vi "WF0_RLE_griffin.vi"(0 "connection ID in":refnum<k5>, 1 "TxPulseRleA":string, 2 "Mode control":enum32{"D-mode", "B-mode"}(ring), 3 "Timeout (ms)":i32=40000000, 4 "TxFrequencyIndex":i8) -> (5 "connection ID out":refnum<k5>, 7 "Timeout (ms) out":i32)   [LabVIEW 2016]
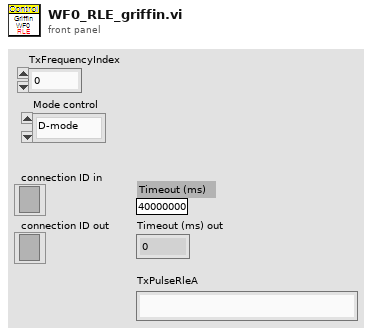
[diagram p1: front panel]
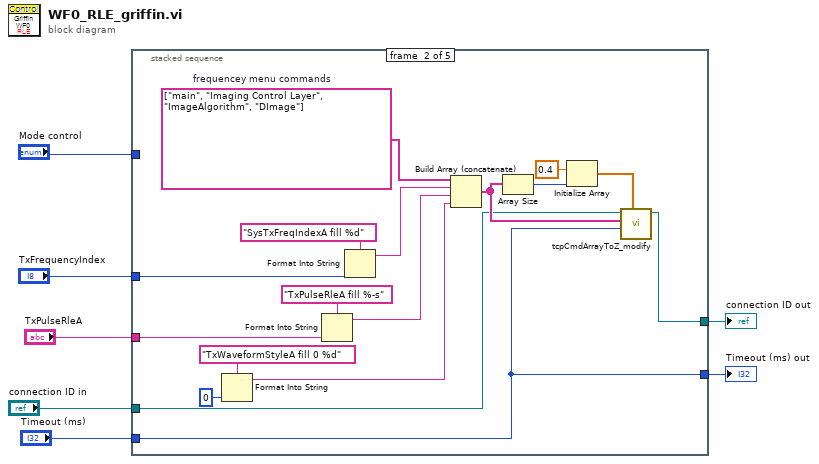
[diagram p0: block diagram]
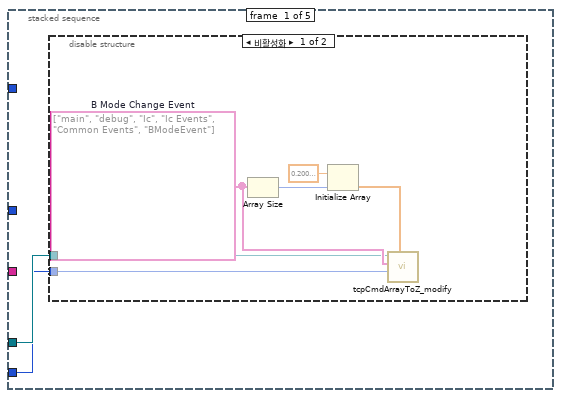
[diagram p2: hidden frame]
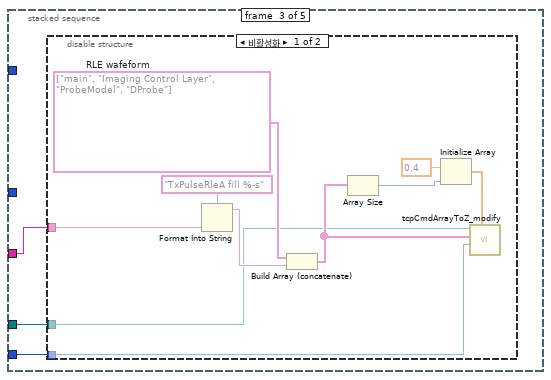
[diagram p4: hidden frame]
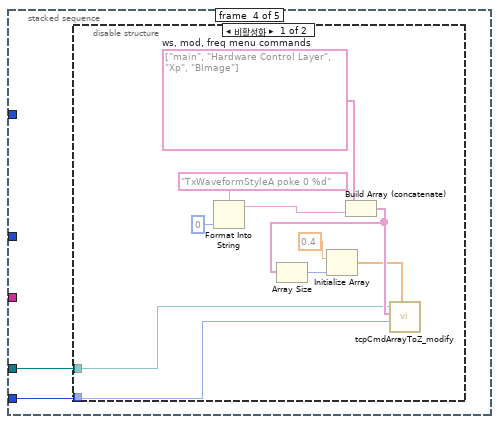
[diagram p6: hidden frame]
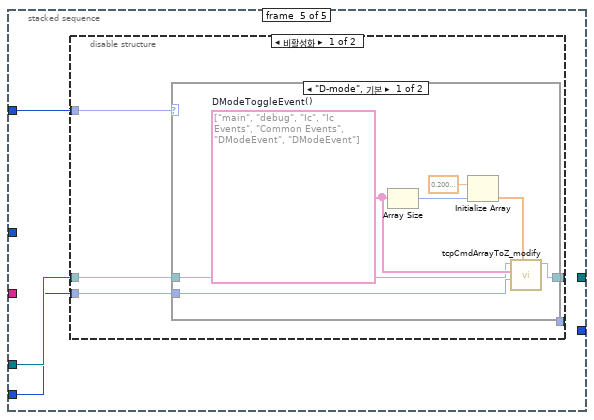
[diagram p8: hidden frame]
diagram:
  n1 = stacked-sequence {
    tunnel: "connection ID in" -> [w9 w25 w34 w47 w60]
    tunnel: "Timeout (ms)" -> [w8 w16 w33 w46 w58]
    tunnel: [_ w17 _ _ _] -> w5
    tunnel: [_ w16 _ _ _] -> w4
    tunnel: "TxPulseRleA" -> [_ w22 w35 _ _]
    tunnel: "Mode control" -> [_ _ _ _ w59]
    tunnel: "TxFrequencyIndex" -> [_ w24 _ _ _]
    frame #0 {
      n2 = disable-structure shown="비활성화" {
        disable-tunnel: w9 -> [w11 _]
        disable-tunnel: w8 -> [w10 _]
        frame Disabled {
          w15 = string[] ["main", "debug", "Ic", "Ic Events", "Common Events", "BModeEvent"]  # B Mode Change Event
          n3 = Array Size(array=w15) -> (size(s)=w12:i32)
          n4 = Initialize Array(sgl 0.2 ("element"), w12) -> (w14:sgl[])
          n5 = call "tcpCmdArrayToZ_modify.vi"("Delay (sec)"=w14, "Timeout (ms)"=w10, "Command array"=w15, "connection ID in"=w11) -> ()  [unwired: 3 in, 5 out]
        }
        frame Enabled {
        }
      }
    }
    frame #1 {
      w28 = string[] ["main", "Imaging Control Layer", "ImageAlgorithm", "DImage"]  # frequencey menu commands
      n6 = Format Into String(format string="TxWaveformStyleA fill 0 %d" ("Format String"), i8 0 ("입력 1")) -> (resulting string=w18:string)  [unwired: 2 in, 1 out]
      n7 = Format Into String(format string="TxPulseRleA fill %-s" ("Format String"), w22) -> (resulting string=w21:string)  [unwired: 2 in, 1 out]
      n8 = Format Into String(format string="SysTxFreqIndexA fill %d" ("초기 문자열"), w24) -> (resulting string=w29:string)  [unwired: 2 in, 1 out]
      n9 = Build Array (concatenate)(w28, w29, w21, w18) -> (w26:string[])
      n10 = Array Size(array=w26) -> (size(s)=w31:i32)
      n11 = Initialize Array(0.4 ("원소"), w31) -> (w30:dbl[])
      n12 = call "tcpCmdArrayToZ_modify.vi"("Delay (sec)"=w30, "Timeout (ms)"=w16, "Command array"=w26, "connection ID in"=w25) -> ("connection ID out"=w17:refnum<k5>)  [unwired: 3 in, 4 out]
    }
    frame #2 {
      n13 = disable-structure shown="비활성화" {
        disable-tunnel: w35 -> [w38 _]
        disable-tunnel: w34 -> [w37 _]
        disable-tunnel: w33 -> [w36 _]
        frame Disabled {
          w39 = string[] ["main", "Imaging Control Layer", "ProbeModel", "DProbe"]  # RLE wafeform
          n14 = Format Into String(format string="TxPulseRleA fill %-s" ("Format String"), w38) -> (resulting string=w43:string)  [unwired: 2 in, 1 out]
          n15 = Build Array (concatenate)(w39, w43) -> (w44:string[])
          n16 = Array Size(array=w44) -> (size(s)=w45:i32)
          n17 = Initialize Array(0.4 ("element"), w45) -> (w41:dbl[])
          n18 = call "tcpCmdArrayToZ_modify.vi"("Delay (sec)"=w41, "Timeout (ms)"=w36, "Command array"=w44, "connection ID in"=w37) -> ()  [unwired: 3 in, 5 out]
        }
        frame Enabled {
        }
      }
    }
    frame #3 {
      n19 = disable-structure shown="비활성화" {
        disable-tunnel: w47 -> [w50 _]
        disable-tunnel: w46 -> [w49 _]
        frame Disabled {
          w56 = string[] ["main", "Hardware Control Layer", "Xp", "BImage"]  # ws, mod, freq menu commands
          n20 = Format Into String(format string="TxWaveformStyleA poke 0 %d" ("Format String"), i8 0 ("입력 1")) -> (resulting string=w55:string)  [unwired: 2 in, 1 out]
          n21 = Build Array (concatenate)(w56, w55) -> (w54:string[])
          n22 = Array Size(array=w54) -> (size(s)=w53:i32)
          n23 = Initialize Array(0.4 ("원소"), w53) -> (w51:dbl[])
          n24 = call "tcpCmdArrayToZ_modify.vi"("Delay (sec)"=w51, "Timeout (ms)"=w49, "Command array"=w54, "connection ID in"=w50) -> ()  [unwired: 3 in, 5 out]
        }
        frame Enabled {
        }
      }
    }
    frame #4 {
      n25 = disable-structure shown="비활성화" {
        disable-tunnel: [w64 w74] -> _
        disable-tunnel: w58 -> [w63 w73]
        disable-tunnel: w60 -> [w62 w74]
        disable-tunnel: w59 -> [w61 _]
        disable-tunnel: [_ w73] -> _
        frame Disabled {
          n26 = case shown="\"D-mode\", 기본" w61 {
            tunnel: [w67 w72] -> w64
            tunnel: w63 -> [w66 _]
            tunnel: w62 -> [w65 w72]
            frame "D-mode", Default {
              w68 = string[] ["main", "debug", "Ic", "Ic Events", "Common Events", "DModeEvent", "DModeEvent"]  # DModeToggleEvent()
              n27 = Array Size(array=w68) -> (size(s)=w71:i32)
              n28 = Initialize Array(sgl 0.2 ("element"), w71) -> (w69:sgl[])
              n29 = call "tcpCmdArrayToZ_modify.vi"("Delay (sec)"=w69, "Timeout (ms)"=w66, "Command array"=w68, "connection ID in"=w65) -> ("connection ID out"=w67:refnum<k5>)  [unwired: 3 in, 4 out]
            }
            frame "B-mode" {
            }
          }
        }
        frame Enabled {
        }
      }
    }
  }
  "connection ID out" <- w5
  "Timeout (ms) out" <- w4
